vi "Clear.vi"(8 "error in (no error)":errorcluster, 11 "task":T1) -> (0 "error out":errorcluster)   [LabVIEW 2022 SP3, in "Combo Digital Audio API.lvlib"]
uses:
  Combo Digital Audio API.lvlib
  <vilib>/PDM Acquisition Toolkit/host/API/PDM Acquisition Toolkit.lvlib
  <vilib>/PDM Acquisition Toolkit/host/API/Public/Clear/Clear PDM Input Task.vi
  task conversion/DAAG task conversion.lvlib
  task conversion/To PDM task.vi
  <vilib>/PDM Acquisition Toolkit/host/API/Public/Clear/Clear PCM Input Task.vi
  <vilib>/PDM Acquisition Toolkit/host/API/Public/Stop/Stop PCM Input Task.vi
  task conversion/To PCM task.vi
  controls/input type.ctl
  task.ctl
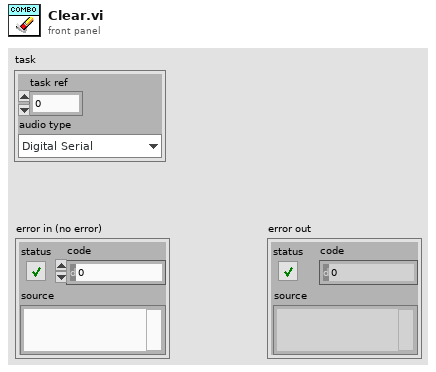
[diagram p1: front panel]
types:
  T1 = typedef "Combo Digital Audio API.lvlib/task.ctl" = cluster{"task ref":u64, "audio type":T2}
  T2 = typedef "input type.ctl" = enum32{"Digital Serial", "PDM"}
  T3 = typedef "PDM Acquisition Class Library.lvlib/PCM Input Task.lvclass/DVR PCM Input Task.ctl" = refnum<data-value>
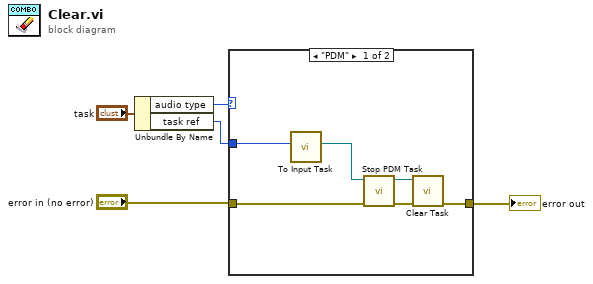
[diagram p0: block diagram]
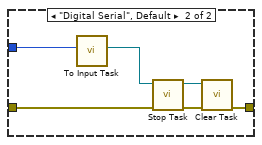
[diagram p2: hidden frame]
diagram:
  n1 = Unbundle By Name("task") -> ("audio type"=w4:T2, "task ref"=w3:u64)
  n2 = case shown="\"PDM\"" w4 {
    tunnel: [w9 w14] -> w1
    tunnel: "error in (no error)" -> [w8 w15]
    tunnel: w3 -> [w7 w13]
    frame "PDM" {
      n3 = call-poly "To Input Task.vi"("task"=w7) -> ("PDM task"=w6:refnum<data-value>)  [unwired: 10 in]
      n4 = call <vilib>:"Stop PDM Task.vi"("error in"=w8, "PDM input task in"=w6) -> ("error out"=w10:errorcluster, "PDM input task out"=w11:refnum<data-value>)  [unwired: 8 in]
      n5 = call-poly <vilib>:"Clear Task.vi"("error in"=w10, "PDM input task in"=w11) -> ("error out"=w9:errorcluster)  [unwired: 9 in]
    }
    frame "Digital Serial", Default {
      n6 = call-poly "To Input Task.vi"("task"=w13) -> ("PCM task"=w12:T3)  [unwired: 10 in]
      n7 = call-poly <vilib>:"Stop Task.vi"("error in"=w15, "PCM input task In"=w12) -> ("error out"=w16:errorcluster, "PCM input task out"=w17:T3)  [unwired: 8 in]
      n8 = call-poly <vilib>:"Clear Task.vi"("error in"=w16, "PCM input task in"=w17) -> ("error out"=w14:errorcluster)  [unwired: 9 in]
    }
  }
  "error out" <- w1
